vi "Autonomous Independent.vi"() -> ()   [LabVIEW 2013]
doc: "This VI is called when autonomous begins, and will automatically be terminated when autonomous ends. You can carry out timed or sensor driven robot movement independently without needing to return to the caller."
uses:
  <vilib>/Rock Robotics/WPI/Relay/WPI_RelayValue.ctl
  Robot Global Data.vi
  <vilib>/Rock Robotics/WPI/RobotDrive/WPI_RobotDriveGetSetRefNum.vi
  <vilib>/addons/control/pid/pid.llb/PID (DBL).vi
  <vilib>/Rock Robotics/WPI/RobotDrive/WPI_RobotDriveMecanumDrive_Cartesian.vi
  <vilib>/Rock Robotics/WPI/Joystick/WPI_JoystickGetSetRefNum.vi
  <vilib>/addons/control/pid/NI_PID_pid.lvlib
panel:
  out "Motor Outputs 2":dbl(graph)=0.07468179223935595
  in  "Target Center Gains":T1={"proportional gain (Kc)"=0.2, "integral time (Ti, min)"=0.0, "derivative time (Td, min)"=0.4} {"derivative time (Td, min)" format="%#.6g"; "integral time (Ti, min)" format="%#.6g"; "proportional gain (Kc)" format="%#.6g"}
  out "Motor Outputs":dbl(graph)=0.07468179223935595
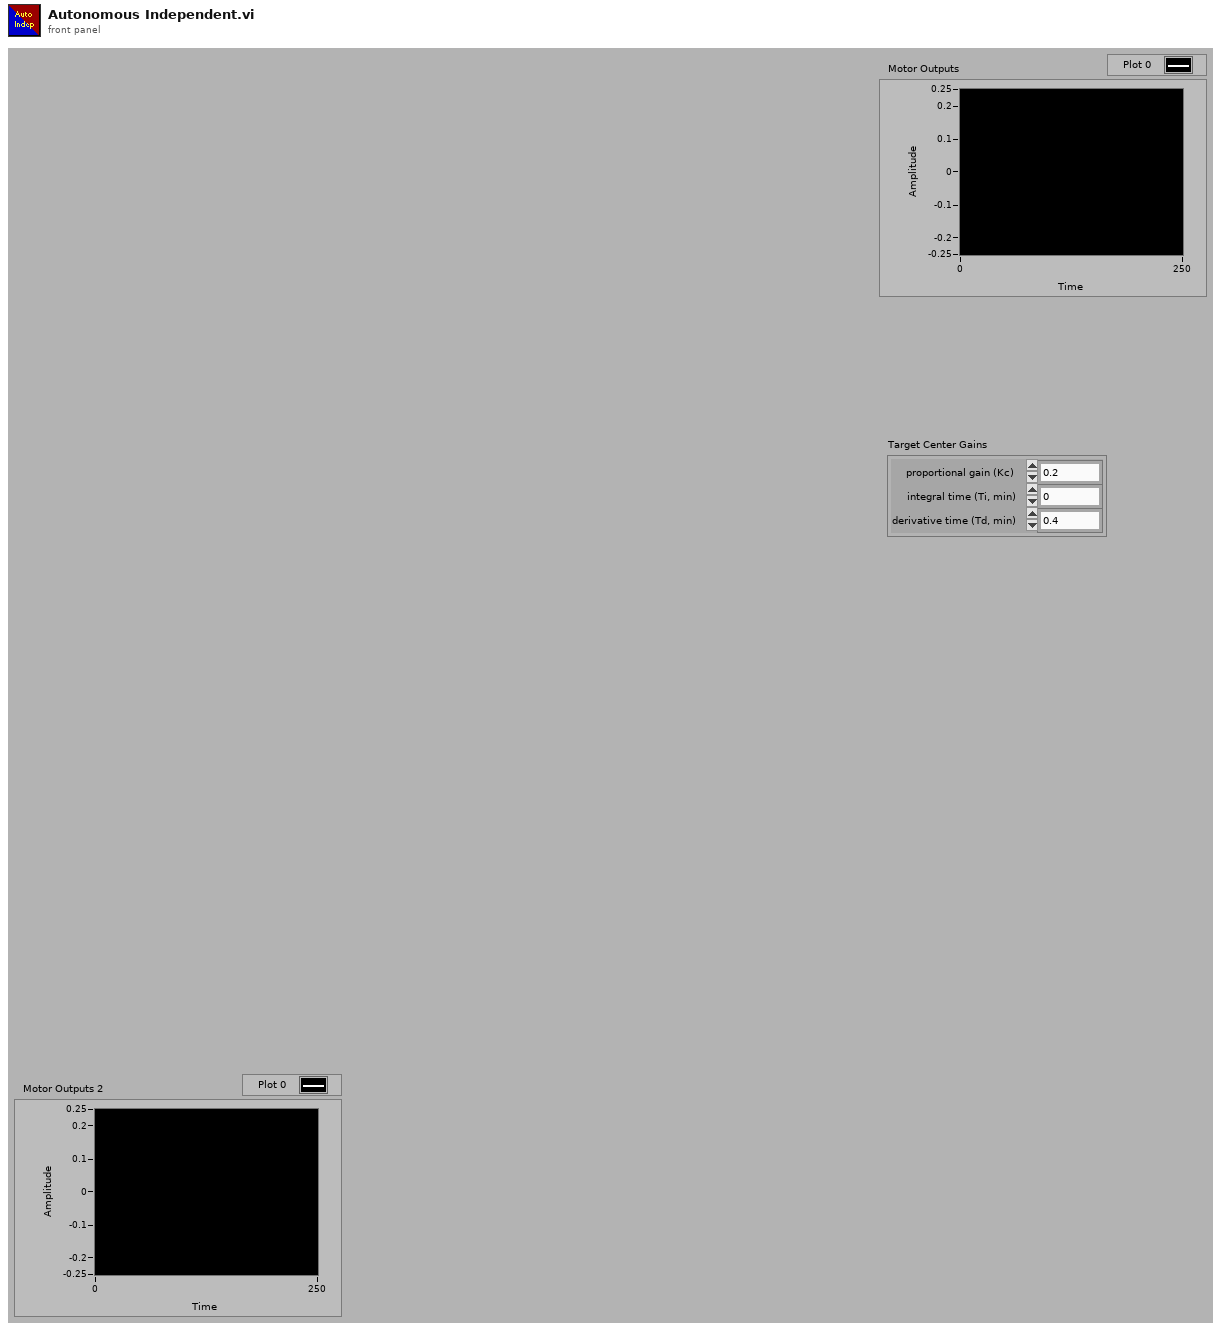
[diagram p1: front panel]
types:
  T1 = cluster{"proportional gain (Kc)":dbl, "integral time (Ti, min)":dbl, "derivative time (Td, min)":dbl}
  T2 = typedef "WPI_RobotDriveDevRef.ctl" = cluster{"DevStatus":errorcluster, "Motors[]":T3[], "Square Inputs":bool, "Max Output":dbl, "Isochronous":bool}
  T3 = typedef "WPI_MotorControlDeviceRef.ctl" = cluster{"DeviceStatus":errorcluster, "Type":enum16{"PWM", "CAN"}, "PWM":cluster{"Digital Module":T4, "PWM Channel":T5, "DeadBand":T6}, "CAN":cluster{"Device Number":u8, "Control Mode":T7, "Semaphore":T8, "Max Vout":dbl}, "Invert":bool, "TransformRef":T9, "InvTransformRef":T9}
  T4 = typedef "FPGA_TypedefDigitalModule.ctl" = enum16{"Digital Module 1", "Digital Module 2"}
  T5 = typedef "FPGA_DIOPWMChannel.ctl" = enum8{"PWM 1", "PWM 2", "PWM 3", "PWM 4", "PWM 5", "PWM 6", "PWM 7", "PWM 8", "PWM 9", "PWM 10", "Invalid"}
  T6 = typedef "WPI_PWMDeadband.ctl" = cluster{"Name":string, "maxPositivePwm":i32, "minPositivePwm":i32, "centerPwm":i32, "maxNegativePwm":i32, "minNegativePwm":i32, "angularRange":u16}
  T7 = typedef "WPI_CANJaguar_ControlMode.ctl" = enum8{"Percent VBus", "Current", "Speed", "Position", "Voltage"}
  T8 = typedef "Semaphore RefNum" = refnum<k1>
  T9 = typedef "WPI_PWMTransform_ConPane.ctl" = refnum<vi>
  T10 = typedef "WPI_JoystickDevRef.ctl" = cluster{"Device":T11}
  T11 = typedef "WPI_JoystickDeviceEnum.ctl" = enum16{"USB 1", "USB 2", "USB 3", "USB 4", "Kinect 1", "Kinect 2"}
  T12 = cluster{"axis 1 (x)":dbl, "axis 2 (y)":dbl, "axis 3 (throttle)":dbl, "axis 4":dbl, "axis 5":dbl, "axis 6":dbl}
  T13 = typedef "WPI_RelayValue.ctl" = enum16{"Off", "On", "Forward", "Reverse"}
  T14 = typedef "WPI_RelayDevRef.ctl" = cluster{"DevStatus":errorcluster, "Relay Channel":T15, "Digital Module":T4, "Relay Direction":T16}
  T15 = typedef "FPGA_DIORelayChannel.ctl" = enum8{"Relay 1", "Relay 2", "Relay 3", "Relay 4", "Relay 5", "Relay 6", "Relay 7", "Relay 8", "Invalid"}
  T16 = typedef "WPI_RelayDirection.ctl" = enum16{"Both directions", "Forward only", "Reverse only"}
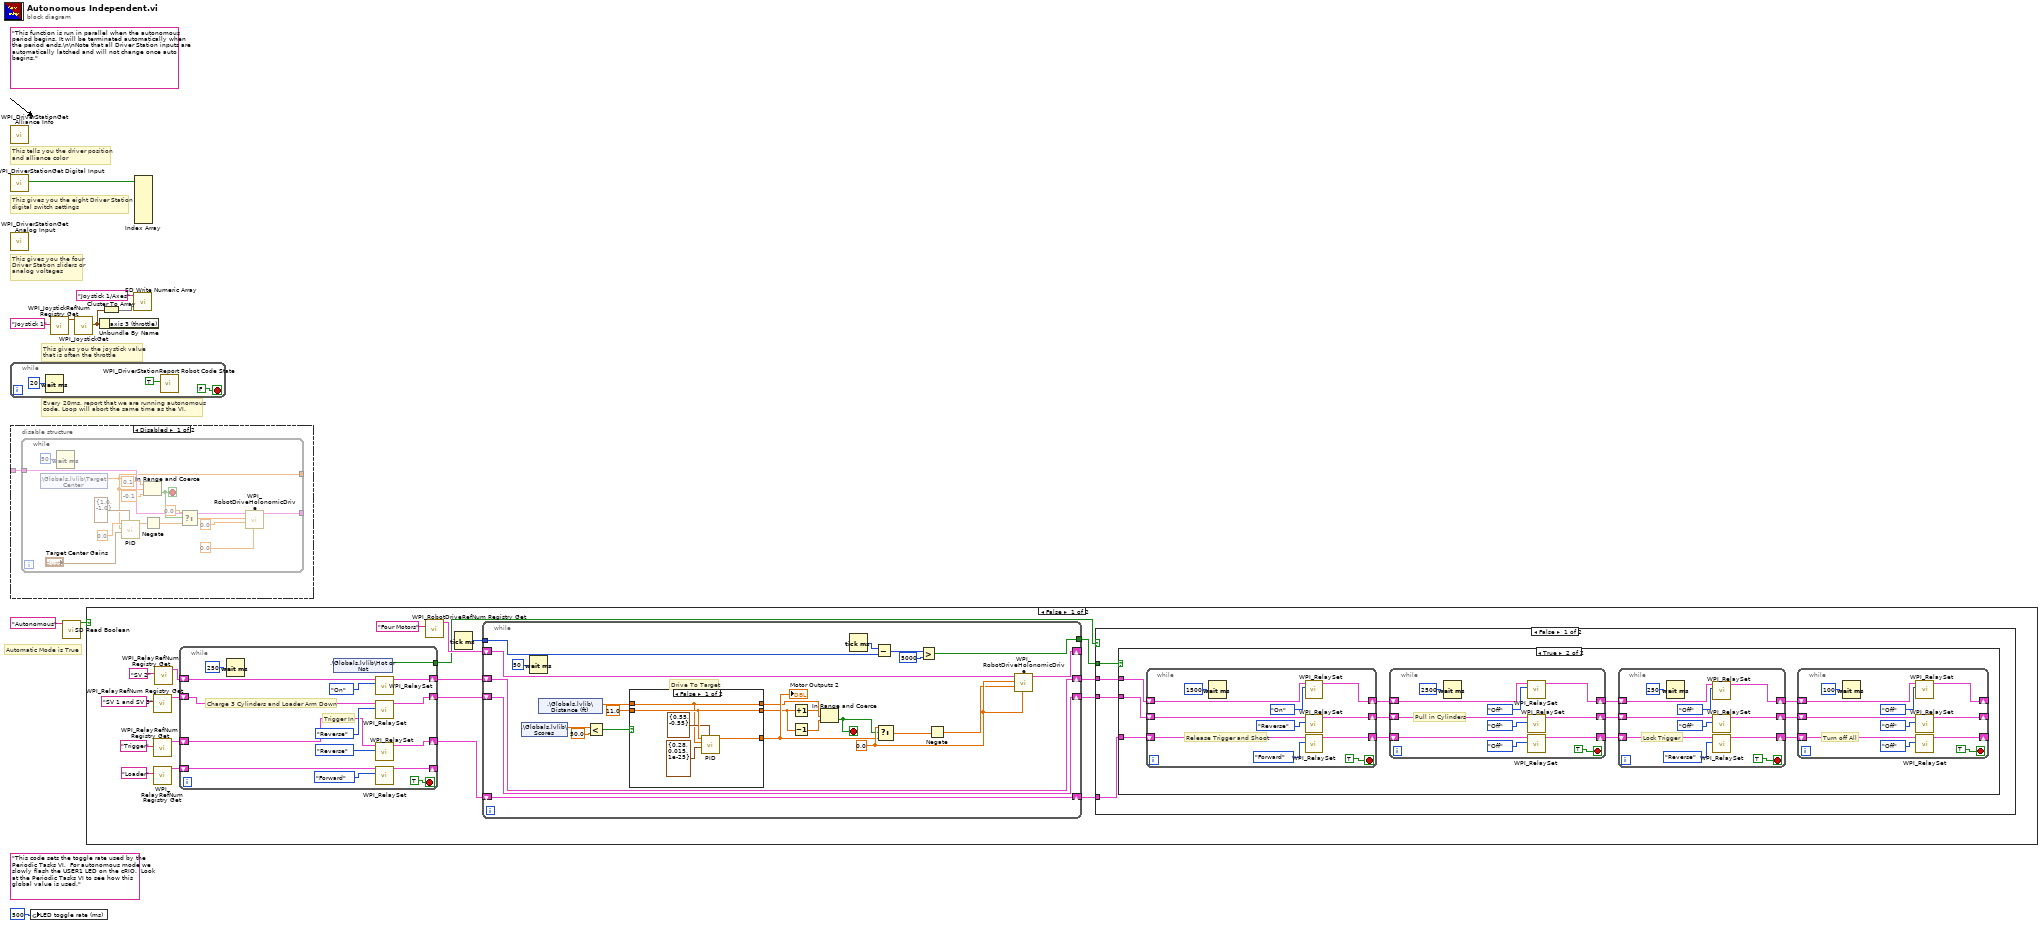
[diagram p0: block diagram]
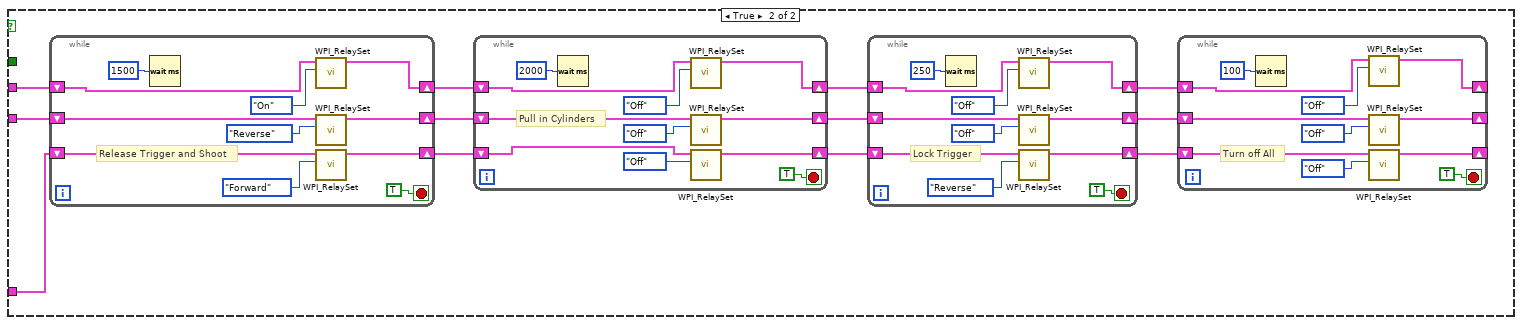
[diagram p3: hidden frame]
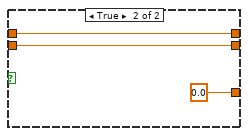
[diagram p4: hidden frame]
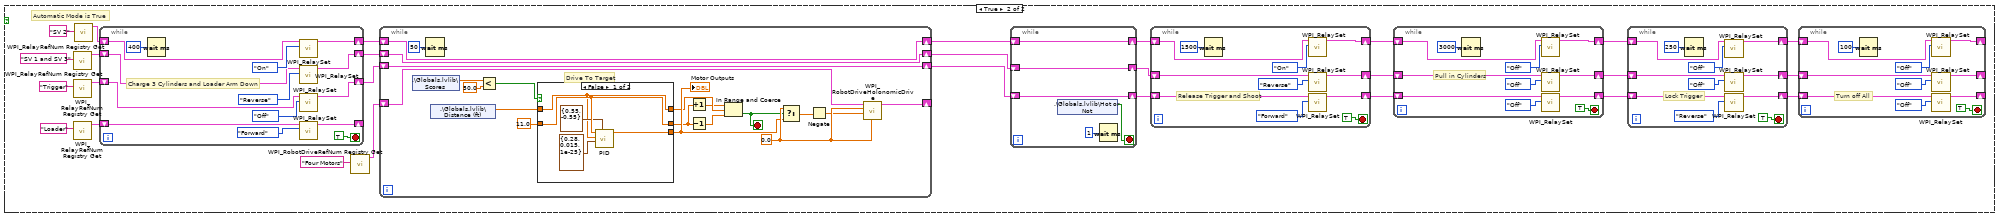
[diagram p5: hidden frame]
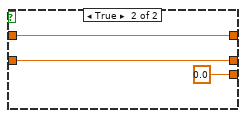
[diagram p6: hidden frame]
diagram:
  (unwired) "This code sets the toggle rate used by the Periodic Tasks VI.  For autonomous mode we slowly flash the USER1 LED on the cRIO.  Look at the Periodic Tasks VI to see how this global value is used."
  (unwired) "This function is run in parallel when the autonomous period begins. It will be terminated automatically when the period ends.\n\nNote that all Driver Station inputs are automatically latched and will not change once auto begins."
  # "Automatic Mode is True"
  # "Every 20ms, report that we are running autonomous\ncode. Loop will abort the same time as the VI."
  # "This gives you the joystick value\nthat is often the throttle"
  # "This tells you the driver position\nand alliance color"
  # "This gives you the eight Driver Station\ndigital switch settings"
  # "This gives you the four\nDriver Station sliders or\nanalog voltages"
  n1 = call <vilib>:"WPI_DriverStationGet Alliance Info.vi"() -> ()  [unwired: 12 out]
  n2 = call <vilib>:"WPI_DriverStationGet Digital Input.vi"() -> ("Driver Station Digital Input (1-8)"=w9:bool[])  [unwired: 11 out]
  n3 = call <vilib>:"WPI_DriverStationGet Analog Input.vi"() -> ()  [unwired: 12 out]
  n4 = while {
    stop <- FALSE stop-if-true
    n5 = Wait (ms)(milliseconds to wait=u32 20) -> ()  [unwired: 1 out]
    n6 = call <vilib>:"WPI_DriverStationReport Robot Code State.vi"("Autonomous"=TRUE) -> ()  [unwired: 10 in, 1 out]
  }
  n7 = disable-structure shown="Disabled" {
    disable-tunnel: _ -> [w13 _]
    frame Disabled {
      n8 = while {
        tunnel: w13 -> [w29]
        tunnel: [w17] -> _
        tunnel: [w16] -> _
        stop <- w15 stop-if-true
        n9 = shared-variable ".\\Globals.lvlib\\Target Center"() -> (w17:dbl)  [unwired: 1 in, 1 out]
        n10 = Wait (ms)(milliseconds to wait=u32 50) -> ()  [unwired: 1 out]
        n11 = call-poly <vilib>:"PID.vi"("output range"=cluster{"output high":dbl, "output low":dbl} {"output high"=1.0, "output low"=-1.0}, "PID gains"="Target Center Gains", "process variable"=w17, "setpoint"=0.0) -> ("output"=w24:dbl)  [unwired: 6 in, 1 out]
        n12 = In Range and Coerce(upper limit=0.1, x=w17, lower limit=-0.1) -> (In Range?=w15:bool)  [unwired: 1 out]
        n13 = Negate(x=w24) -> (-x=w20:dbl)
        n14 = Select(t=0.0, s=w15, f=w20) -> (s? t:f=w19:dbl)
        n15 = call-poly <vilib>:"WPI_RobotDriveHolonomicDrive.vi"("Rotation"=0.0 ("Y"), "Y"=0.0, "X"=w19, "RobotDriveDevRef"=w29) -> ("RobotDriveDevRef"=w16:T2)  [unwired: 5 in, 2 out]
      }
    }
    frame Enabled {
    }
  }
  n16 = global write "Robot Global Data.vi" "LED toggle rate (ms)"(u32 500 ("LED ms toggle rate")) -> ()
  n17 = call <vilib>:"WPI_JoystickRefNum Registry Get.vi"("refnum name"="Joystick 1") -> ("JoystickDevRef"=w7:T10)  [unwired: 1 in, 9 out]
  n18 = call <vilib>:"SD Read Boolean.vi"("Name"="Autonomous") -> ("Boolean"=w1:bool)  [unwired: 8 in, 2 out]
  n19 = call <vilib>:"WPI_JoystickGet.vi"("JoystickDevRef"=w7) -> ("Axes"=w5:T12)  [unwired: 1 in, 5 out]
  n20 = case shown="False" w1 {
    frame False {
      n21 = call <vilib>:"WPI_RelayRefNum Registry Get.vi"("refnum name"="SV 1 and SV 3") -> ("RelayDevRef"=w41:T14)  [unwired: 9 in, 1 out]
      n22 = call <vilib>:"WPI_RelayRefNum Registry Get.vi"("refnum name"="Trigger") -> ("RelayDevRef"=w42:T14)  [unwired: 9 in, 1 out]
      n23 = call <vilib>:"WPI_RelayRefNum Registry Get.vi"("refnum name"="Loader") -> ("RelayDevRef"=w39:T14)  [unwired: 9 in, 1 out]
      n24 = call <vilib>:"WPI_RelayRefNum Registry Get.vi"("refnum name"="SV 2") -> ("RelayDevRef"=w44:T14)  [unwired: 9 in, 1 out]
      n25 = while {
        shift-right: [w172] -> w36
        shift-left: w42 -> [w173]
        shift-right: [w175] -> w38
        shift-left: w44 -> [w176]
        shift-right: [w170] -> w37
        shift-left: w41 -> [w169]
        shift-right: [w166] -> _
        shift-left: w39 -> [w167]
        tunnel: [w165] -> w30
        stop <- TRUE stop-if-true
        # "Trigger In"
        # "Charge 3 Cylinders and Loader Arm Down"
        n26 = Wait (ms)(milliseconds to wait=u32 250) -> ()  [unwired: 1 out]
        n27 = shared-variable ".\\Globals.lvlib\\Hot or Not"() -> (w165:bool)  [unwired: 1 in, 1 out]
        n28 = call <vilib>:"WPI_RelaySet.vi"("RelayValue"=WPI_RelayValue."On", "RelayDevRef"=w176) -> ("RelayDevRef"=w175:T14)  [unwired: 8 in, 1 out]
        n29 = call <vilib>:"WPI_RelaySet.vi"("RelayValue"=WPI_RelayValue."Reverse", "RelayDevRef"=w169) -> ("RelayDevRef"=w170:T14)  [unwired: 8 in, 1 out]
        n30 = call <vilib>:"WPI_RelaySet.vi"("RelayValue"=WPI_RelayValue."Reverse", "RelayDevRef"=w173) -> ("RelayDevRef"=w172:T14)  [unwired: 8 in, 1 out]
        n31 = call <vilib>:"WPI_RelaySet.vi"("RelayValue"=WPI_RelayValue."Forward", "RelayDevRef"=w167) -> ("RelayDevRef"=w166:T14)  [unwired: 8 in, 1 out]
      }
      n32 = call <vilib>:"WPI_RobotDriveRefNum Registry Get.vi"("refnum name"="Four Motors") -> ("RobotDriveDevRef"=w47:T2)  [unwired: 1 in, 9 out]
      n33 = Tick Count (ms)() -> (millisecond timer value=w32:u32)
      n34 = while {
        shift-right: [w199] -> _
        shift-left: w47 -> [w204]
        shift-right: [w187] -> w33
        shift-left: w36 -> [w187]
        shift-right: [w186] -> w35
        shift-left: w38 -> [w186]
        shift-right: [w185] -> w34
        shift-left: w37 -> [w185]
        tunnel: w32 -> [w181]
        tunnel: [w180] -> w31
        stop <- w192 stop-if-true
        w196 = 0.0 ("output")
        # "Drive To Target"
        n35 = shared-variable ".\\Globals.lvlib\\Scores"() -> (w203:dbl)  [unwired: 1 in, 1 out]
        n36 = Wait (ms)(milliseconds to wait=u32 50) -> ()  [unwired: 1 out]
        n37 = shared-variable ".\\Globals.lvlib\\Distance (ft)"() -> (w194:dbl)  [unwired: 1 in, 1 out]
        n38 = Less?(x=w203, y=50.0) -> (x < y?=w201:bool)
        n39 = case shown="False" w201 {
          tunnel: [w209 w212] -> w191
          tunnel: 11.0 ("setpoint") -> [w209 w212]
          tunnel: [w207 0.0 ("output")] -> w195
          tunnel: w194 -> [w205 w210]
          tunnel: [w205 w210] -> w193
          frame False {
            n40 = call-poly <vilib>:"PID.vi"("output range"=cluster{"output high":dbl, "output low":dbl} {"output high"=0.55, "output low"=-0.55}, "PID gains"=T1 {"proportional gain (Kc)"=0.28, "integral time (Ti, min)"=0.015, "derivative time (Td, min)"=1e-25} ("Distance Gains"), "process variable"=w205, "setpoint"=w209) -> ("output"=w207:dbl)  [unwired: 6 in, 1 out]
          }
          frame True {
          }
        }
        "Motor Outputs 2" <- w195
        n41 = Increment(x=w191) -> (x+1=w190:dbl)
        n42 = Decrement(x=w191) -> (x-1=w200:dbl)
        n43 = In Range and Coerce(upper limit=w190, x=w193, lower limit=w200) -> (In Range?=w192:bool)  [unwired: 1 out]
        n44 = Tick Count (ms)() -> (millisecond timer value=w184:u32)
        n45 = Subtract(x=w184, y=w181) -> (x-y=w182:u32)
        n46 = Select(t=w196, s=w192, f=w195) -> (s? t:f=w189:dbl)
        n47 = Greater?(x=w182, y=u32 5000) -> (0:w180:bool)
        n48 = Negate(x=w189) -> (-x=w188:dbl)
        n49 = call-poly <vilib>:"WPI_RobotDriveHolonomicDrive.vi"("Rotation"=w196, "Y"=w188, "X"=w196, "RobotDriveDevRef"=w204) -> ("RobotDriveDevRef"=w199:T2)  [unwired: 5 in, 2 out]
      }
      n50 = case shown="False" w30 {
        tunnel: w35 -> [w51 w111]
        tunnel: w34 -> [w50 w110]
        tunnel: w33 -> [w49 w109]
        tunnel: w31 -> [w52 _]
        frame False {
          n51 = case shown="True" w52 {
            tunnel: w51 -> [_ w55]
            tunnel: w50 -> [_ w54]
            tunnel: w49 -> [_ w53]
            frame False {
            }
            frame True {
              n52 = while {
                shift-right: [w83] -> w63
                shift-left: w53 -> [w84]
                shift-right: [w78] -> w62
                shift-left: w55 -> [w79]
                shift-right: [w80] -> w61
                shift-left: w54 -> [w81]
                stop <- TRUE stop-if-true
                # "Release Trigger and Shoot"
                n53 = Wait (ms)(milliseconds to wait=u32 1500) -> ()  [unwired: 1 out]
                n54 = call <vilib>:"WPI_RelaySet.vi"("RelayValue"=WPI_RelayValue."On", "RelayDevRef"=w79) -> ("RelayDevRef"=w78:T14)  [unwired: 8 in, 1 out]
                n55 = call <vilib>:"WPI_RelaySet.vi"("RelayValue"=WPI_RelayValue."Reverse", "RelayDevRef"=w81) -> ("RelayDevRef"=w80:T14)  [unwired: 8 in, 1 out]
                n56 = call <vilib>:"WPI_RelaySet.vi"("RelayValue"=WPI_RelayValue."Forward", "RelayDevRef"=w84) -> ("RelayDevRef"=w83:T14)  [unwired: 8 in, 1 out]
              }
              n57 = while {
                shift-right: [w93] -> w59
                shift-left: w62 -> [w94]
                shift-right: [w88] -> w64
                shift-left: w63 -> [w89]
                shift-right: [w91] -> w60
                shift-left: w61 -> [w92]
                stop <- TRUE stop-if-true
                # "Pull in Cylinders"
                n58 = Wait (ms)(milliseconds to wait=u32 2500) -> ()  [unwired: 1 out]
                n59 = call <vilib>:"WPI_RelaySet.vi"("RelayValue"=WPI_RelayValue."Off", "RelayDevRef"=w94) -> ("RelayDevRef"=w93:T14)  [unwired: 8 in, 1 out]
                n60 = call <vilib>:"WPI_RelaySet.vi"("RelayValue"=WPI_RelayValue."Off", "RelayDevRef"=w92) -> ("RelayDevRef"=w91:T14)  [unwired: 8 in, 1 out]
                n61 = call <vilib>:"WPI_RelaySet.vi"("RelayValue"=WPI_RelayValue."Off", "RelayDevRef"=w89) -> ("RelayDevRef"=w88:T14)  [unwired: 8 in, 1 out]
              }
              n62 = while {
                shift-right: [w105] -> w57
                shift-left: w64 -> [w106]
                shift-right: [w102] -> w56
                shift-left: w59 -> [w103]
                shift-right: [w100] -> w58
                shift-left: w60 -> [w101]
                stop <- TRUE stop-if-true
                # "Lock Trigger"
                n63 = Wait (ms)(milliseconds to wait=u32 250) -> ()  [unwired: 1 out]
                n64 = call <vilib>:"WPI_RelaySet.vi"("RelayValue"=WPI_RelayValue."Off", "RelayDevRef"=w103) -> ("RelayDevRef"=w102:T14)  [unwired: 8 in, 1 out]
                n65 = call <vilib>:"WPI_RelaySet.vi"("RelayValue"=WPI_RelayValue."Off", "RelayDevRef"=w101) -> ("RelayDevRef"=w100:T14)  [unwired: 8 in, 1 out]
                n66 = call <vilib>:"WPI_RelaySet.vi"("RelayValue"=WPI_RelayValue."Reverse", "RelayDevRef"=w106) -> ("RelayDevRef"=w105:T14)  [unwired: 8 in, 1 out]
              }
              n67 = while {
                shift-right: [w72] -> _
                shift-left: w57 -> [w73]
                shift-right: [w69] -> _
                shift-left: w56 -> [w70]
                shift-right: [w67] -> _
                shift-left: w58 -> [w68]
                stop <- TRUE stop-if-true
                # "Turn off All"
                n68 = Wait (ms)(milliseconds to wait=u32 100) -> ()  [unwired: 1 out]
                n69 = call <vilib>:"WPI_RelaySet.vi"("RelayValue"=WPI_RelayValue."Off", "RelayDevRef"=w70) -> ("RelayDevRef"=w69:T14)  [unwired: 8 in, 1 out]
                n70 = call <vilib>:"WPI_RelaySet.vi"("RelayValue"=WPI_RelayValue."Off", "RelayDevRef"=w68) -> ("RelayDevRef"=w67:T14)  [unwired: 8 in, 1 out]
                n71 = call <vilib>:"WPI_RelaySet.vi"("RelayValue"=WPI_RelayValue."Off", "RelayDevRef"=w73) -> ("RelayDevRef"=w72:T14)  [unwired: 8 in, 1 out]
              }
            }
          }
        }
        frame True {
          n72 = while {
            shift-right: [w139] -> w119
            shift-left: w109 -> [w140]
            shift-right: [w134] -> w118
            shift-left: w111 -> [w135]
            shift-right: [w136] -> w117
            shift-left: w110 -> [w137]
            stop <- TRUE stop-if-true
            # "Release Trigger and Shoot"
            n73 = Wait (ms)(milliseconds to wait=u32 1500) -> ()  [unwired: 1 out]
            n74 = call <vilib>:"WPI_RelaySet.vi"("RelayValue"=WPI_RelayValue."On", "RelayDevRef"=w135) -> ("RelayDevRef"=w134:T14)  [unwired: 8 in, 1 out]
            n75 = call <vilib>:"WPI_RelaySet.vi"("RelayValue"=WPI_RelayValue."Reverse", "RelayDevRef"=w137) -> ("RelayDevRef"=w136:T14)  [unwired: 8 in, 1 out]
            n76 = call <vilib>:"WPI_RelaySet.vi"("RelayValue"=WPI_RelayValue."Forward", "RelayDevRef"=w140) -> ("RelayDevRef"=w139:T14)  [unwired: 8 in, 1 out]
          }
          n77 = while {
            shift-right: [w149] -> w115
            shift-left: w118 -> [w150]
            shift-right: [w144] -> w120
            shift-left: w119 -> [w145]
            shift-right: [w147] -> w116
            shift-left: w117 -> [w148]
            stop <- TRUE stop-if-true
            # "Pull in Cylinders"
            n78 = Wait (ms)(milliseconds to wait=u32 2000) -> ()  [unwired: 1 out]
            n79 = call <vilib>:"WPI_RelaySet.vi"("RelayValue"=WPI_RelayValue."Off", "RelayDevRef"=w150) -> ("RelayDevRef"=w149:T14)  [unwired: 8 in, 1 out]
            n80 = call <vilib>:"WPI_RelaySet.vi"("RelayValue"=WPI_RelayValue."Off", "RelayDevRef"=w148) -> ("RelayDevRef"=w147:T14)  [unwired: 8 in, 1 out]
            n81 = call <vilib>:"WPI_RelaySet.vi"("RelayValue"=WPI_RelayValue."Off", "RelayDevRef"=w145) -> ("RelayDevRef"=w144:T14)  [unwired: 8 in, 1 out]
          }
          n82 = while {
            shift-right: [w161] -> w113
            shift-left: w120 -> [w162]
            shift-right: [w158] -> w112
            shift-left: w115 -> [w159]
            shift-right: [w156] -> w114
            shift-left: w116 -> [w157]
            stop <- TRUE stop-if-true
            # "Lock Trigger"
            n83 = Wait (ms)(milliseconds to wait=u32 250) -> ()  [unwired: 1 out]
            n84 = call <vilib>:"WPI_RelaySet.vi"("RelayValue"=WPI_RelayValue."Off", "RelayDevRef"=w159) -> ("RelayDevRef"=w158:T14)  [unwired: 8 in, 1 out]
            n85 = call <vilib>:"WPI_RelaySet.vi"("RelayValue"=WPI_RelayValue."Off", "RelayDevRef"=w157) -> ("RelayDevRef"=w156:T14)  [unwired: 8 in, 1 out]
            n86 = call <vilib>:"WPI_RelaySet.vi"("RelayValue"=WPI_RelayValue."Reverse", "RelayDevRef"=w162) -> ("RelayDevRef"=w161:T14)  [unwired: 8 in, 1 out]
          }
          n87 = while {
            shift-right: [w128] -> _
            shift-left: w113 -> [w129]
            shift-right: [w125] -> _
            shift-left: w112 -> [w126]
            shift-right: [w123] -> _
            shift-left: w114 -> [w124]
            stop <- TRUE stop-if-true
            # "Turn off All"
            n88 = Wait (ms)(milliseconds to wait=u32 100) -> ()  [unwired: 1 out]
            n89 = call <vilib>:"WPI_RelaySet.vi"("RelayValue"=WPI_RelayValue."Off", "RelayDevRef"=w126) -> ("RelayDevRef"=w125:T14)  [unwired: 8 in, 1 out]
            n90 = call <vilib>:"WPI_RelaySet.vi"("RelayValue"=WPI_RelayValue."Off", "RelayDevRef"=w124) -> ("RelayDevRef"=w123:T14)  [unwired: 8 in, 1 out]
            n91 = call <vilib>:"WPI_RelaySet.vi"("RelayValue"=WPI_RelayValue."Off", "RelayDevRef"=w129) -> ("RelayDevRef"=w128:T14)  [unwired: 8 in, 1 out]
          }
        }
      }
    }
    frame True {
      # "Automatic Mode is True"
      n92 = call <vilib>:"WPI_RelayRefNum Registry Get.vi"("refnum name"="SV 1 and SV 3") -> ("RelayDevRef"=w215:T14)  [unwired: 9 in, 1 out]
      n93 = call <vilib>:"WPI_RelayRefNum Registry Get.vi"("refnum name"="Trigger") -> ("RelayDevRef"=w236:T14)  [unwired: 9 in, 1 out]
      n94 = call <vilib>:"WPI_RelayRefNum Registry Get.vi"("refnum name"="Loader") -> ("RelayDevRef"=w213:T14)  [unwired: 9 in, 1 out]
      n95 = call <vilib>:"WPI_RelayRefNum Registry Get.vi"("refnum name"="SV 2") -> ("RelayDevRef"=w238:T14)  [unwired: 9 in, 1 out]
      n96 = while {
        shift-right: [w324] -> w224
        shift-left: w236 -> [w325]
        shift-right: [w327] -> w223
        shift-left: w238 -> [w328]
        shift-right: [w322] -> w222
        shift-left: w215 -> [w321]
        shift-right: [w318] -> _
        shift-left: w213 -> [w319]
        stop <- TRUE stop-if-true
        # "Charge 3 Cylinders and Loader Arm Down"
        n97 = Wait (ms)(milliseconds to wait=u32 400) -> ()  [unwired: 1 out]
        n98 = call <vilib>:"WPI_RelaySet.vi"("RelayValue"=WPI_RelayValue."On", "RelayDevRef"=w328) -> ("RelayDevRef"=w327:T14)  [unwired: 8 in, 1 out]
        n99 = call <vilib>:"WPI_RelaySet.vi"("RelayValue"=WPI_RelayValue."Reverse", "RelayDevRef"=w321) -> ("RelayDevRef"=w322:T14)  [unwired: 8 in, 1 out]
        n100 = call <vilib>:"WPI_RelaySet.vi"("RelayValue"=WPI_RelayValue."Off", "RelayDevRef"=w325) -> ("RelayDevRef"=w324:T14)  [unwired: 8 in, 1 out]
        n101 = call <vilib>:"WPI_RelaySet.vi"("RelayValue"=WPI_RelayValue."Forward", "RelayDevRef"=w319) -> ("RelayDevRef"=w318:T14)  [unwired: 8 in, 1 out]
      }
      n102 = call <vilib>:"WPI_RobotDriveRefNum Registry Get.vi"("refnum name"="Four Motors") -> ("RobotDriveDevRef"=w225:T2)  [unwired: 1 in, 9 out]
      n103 = while {
        shift-right: [w260] -> _
        shift-left: w225 -> [w265]
        shift-right: [w248] -> w219
        shift-left: w224 -> [w248]
        shift-right: [w247] -> w220
        shift-left: w223 -> [w247]
        shift-right: [w246] -> w221
        shift-left: w222 -> [w246]
        stop <- w253 stop-if-true
        w257 = 0.0 ("output")
        # "Drive To Target"
        n104 = shared-variable ".\\Globals.lvlib\\Scores"() -> (w264:dbl)  [unwired: 1 in, 1 out]
        n105 = Wait (ms)(milliseconds to wait=u32 50) -> ()  [unwired: 1 out]
        n106 = shared-variable ".\\Globals.lvlib\\Distance (ft)"() -> (w255:dbl)  [unwired: 1 in, 1 out]
        n107 = Less?(x=w264, y=50.0) -> (x < y?=w262:bool)
        n108 = case shown="False" w262 {
          tunnel: [w270 w273] -> w252
          tunnel: 11.0 ("setpoint") -> [w270 w273]
          tunnel: [w268 0.0 ("output")] -> w256
          tunnel: w255 -> [w266 w271]
          tunnel: [w266 w271] -> w254
          frame False {
            n109 = call-poly <vilib>:"PID.vi"("output range"=cluster{"output high":dbl, "output low":dbl} {"output high"=0.55, "output low"=-0.55}, "PID gains"=T1 {"proportional gain (Kc)"=0.28, "integral time (Ti, min)"=0.015, "derivative time (Td, min)"=1e-25} ("Distance Gains"), "process variable"=w266, "setpoint"=w270) -> ("output"=w268:dbl)  [unwired: 6 in, 1 out]
          }
          frame True {
          }
        }
        "Motor Outputs" <- w256
        n110 = Increment(x=w252) -> (x+1=w251:dbl)
        n111 = Decrement(x=w252) -> (x-1=w261:dbl)
        n112 = In Range and Coerce(upper limit=w251, x=w254, lower limit=w261) -> (In Range?=w253:bool)  [unwired: 1 out]
        n113 = Select(t=w257, s=w253, f=w256) -> (s? t:f=w250:dbl)
        n114 = Negate(x=w250) -> (-x=w249:dbl)
        n115 = call-poly <vilib>:"WPI_RobotDriveHolonomicDrive.vi"("Rotation"=w257, "Y"=w249, "X"=w257, "RobotDriveDevRef"=w265) -> ("RobotDriveDevRef"=w260:T2)  [unwired: 5 in, 2 out]
      }
      n116 = while {
        shift-right: [w243] -> w218
        shift-left: w221 -> [w243]
        shift-right: [w242] -> w217
        shift-left: w220 -> [w242]
        shift-right: [w241] -> w216
        shift-left: w219 -> [w241]
        stop <- w244 stop-if-true
        n117 = shared-variable ".\\Globals.lvlib\\Hot or Not"() -> (w244:bool)  [unwired: 1 in, 1 out]
        n118 = Wait (ms)(milliseconds to wait=u32 1) -> ()  [unwired: 1 out]
      }
      n119 = while {
        shift-right: [w292] -> w234
        shift-left: w216 -> [w293]
        shift-right: [w287] -> w233
        shift-left: w217 -> [w288]
        shift-right: [w289] -> w232
        shift-left: w218 -> [w290]
        stop <- TRUE stop-if-true
        # "Release Trigger and Shoot"
        n120 = Wait (ms)(milliseconds to wait=u32 1500) -> ()  [unwired: 1 out]
        n121 = call <vilib>:"WPI_RelaySet.vi"("RelayValue"=WPI_RelayValue."On", "RelayDevRef"=w288) -> ("RelayDevRef"=w287:T14)  [unwired: 8 in, 1 out]
        n122 = call <vilib>:"WPI_RelaySet.vi"("RelayValue"=WPI_RelayValue."Reverse", "RelayDevRef"=w290) -> ("RelayDevRef"=w289:T14)  [unwired: 8 in, 1 out]
        n123 = call <vilib>:"WPI_RelaySet.vi"("RelayValue"=WPI_RelayValue."Forward", "RelayDevRef"=w293) -> ("RelayDevRef"=w292:T14)  [unwired: 8 in, 1 out]
      }
      n124 = while {
        shift-right: [w302] -> w230
        shift-left: w233 -> [w303]
        shift-right: [w297] -> w235
        shift-left: w234 -> [w298]
        shift-right: [w300] -> w231
        shift-left: w232 -> [w301]
        stop <- TRUE stop-if-true
        # "Pull in Cylinders"
        n125 = Wait (ms)(milliseconds to wait=u32 3000) -> ()  [unwired: 1 out]
        n126 = call <vilib>:"WPI_RelaySet.vi"("RelayValue"=WPI_RelayValue."Off", "RelayDevRef"=w303) -> ("RelayDevRef"=w302:T14)  [unwired: 8 in, 1 out]
        n127 = call <vilib>:"WPI_RelaySet.vi"("RelayValue"=WPI_RelayValue."Off", "RelayDevRef"=w301) -> ("RelayDevRef"=w300:T14)  [unwired: 8 in, 1 out]
        n128 = call <vilib>:"WPI_RelaySet.vi"("RelayValue"=WPI_RelayValue."Off", "RelayDevRef"=w298) -> ("RelayDevRef"=w297:T14)  [unwired: 8 in, 1 out]
      }
      n129 = while {
        shift-right: [w314] -> w228
        shift-left: w235 -> [w315]
        shift-right: [w311] -> w227
        shift-left: w230 -> [w312]
        shift-right: [w309] -> w229
        shift-left: w231 -> [w310]
        stop <- TRUE stop-if-true
        # "Lock Trigger"
        n130 = Wait (ms)(milliseconds to wait=u32 250) -> ()  [unwired: 1 out]
        n131 = call <vilib>:"WPI_RelaySet.vi"("RelayValue"=WPI_RelayValue."Off", "RelayDevRef"=w312) -> ("RelayDevRef"=w311:T14)  [unwired: 8 in, 1 out]
        n132 = call <vilib>:"WPI_RelaySet.vi"("RelayValue"=WPI_RelayValue."Off", "RelayDevRef"=w310) -> ("RelayDevRef"=w309:T14)  [unwired: 8 in, 1 out]
        n133 = call <vilib>:"WPI_RelaySet.vi"("RelayValue"=WPI_RelayValue."Reverse", "RelayDevRef"=w315) -> ("RelayDevRef"=w314:T14)  [unwired: 8 in, 1 out]
      }
      n134 = while {
        shift-right: [w281] -> _
        shift-left: w228 -> [w282]
        shift-right: [w278] -> _
        shift-left: w227 -> [w279]
        shift-right: [w276] -> _
        shift-left: w229 -> [w277]
        stop <- TRUE stop-if-true
        # "Turn off All"
        n135 = Wait (ms)(milliseconds to wait=u32 100) -> ()  [unwired: 1 out]
        n136 = call <vilib>:"WPI_RelaySet.vi"("RelayValue"=WPI_RelayValue."Off", "RelayDevRef"=w279) -> ("RelayDevRef"=w278:T14)  [unwired: 8 in, 1 out]
        n137 = call <vilib>:"WPI_RelaySet.vi"("RelayValue"=WPI_RelayValue."Off", "RelayDevRef"=w277) -> ("RelayDevRef"=w276:T14)  [unwired: 8 in, 1 out]
        n138 = call <vilib>:"WPI_RelaySet.vi"("RelayValue"=WPI_RelayValue."Off", "RelayDevRef"=w282) -> ("RelayDevRef"=w281:T14)  [unwired: 8 in, 1 out]
      }
    }
  }
  n139 = Unbundle By Name(w5) -> ()  [unwired: 1 out]
  n140 = Cluster To Array(cluster=w5) -> (array=w6:dbl[])
  n141 = call <vilib>:"SD Write Numeric Array.vi"("Numeric Array"=w6, "Name"="Joystick 1/Axes") -> ()  [unwired: 8 in, 2 out]
  n142 = Index Array(array=w9) -> ()  [unwired: 8 in, 8 out]
